vi "Level_3.vi"(8 "error in (no error)":errorcluster) -> (0 "error out":errorcluster)   [LabVIEW 2020]
uses:
  classes/Test/Test.lvclass
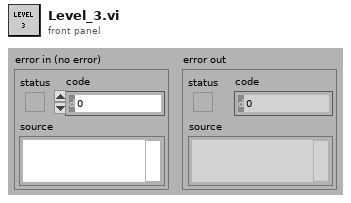
[diagram p1: front panel]
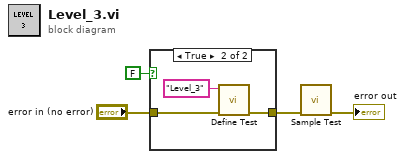
[diagram p0: block diagram]
diagram:
  n1 = case shown="True" FALSE {
    tunnel: "error in (no error)" -> [w5 w7]
    tunnel: [w5 w6] -> w2
    frame False {
    }
    frame True {
      n2 = call "Define Test.vi"("error in (no error)"=w7, "Label (VI Title)"="Level_3") -> ("error out"=w6:errorcluster)  [unwired: 8 in, 1 out]
    }
  }
  n3 = call "Sample Test.vi"("error in (no error)"=w2) -> ("error out"=→"error out":errorcluster)  [unwired: 10 in]
